vi "Create From String.vi"(8 "error in":errorcluster, 10 "Input String":string) -> (0 "error out":errorcluster, 3 "Orient3d out":refnum<class "Orient3d Class.lvclass">)   [LabVIEW 2011, in "Orient3d Class.lvclass"]
uses:
  Orient3d Class.lvclass
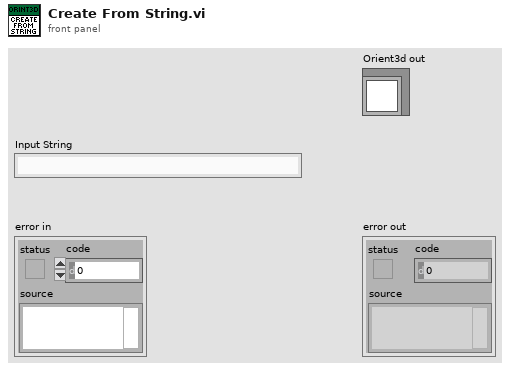
[diagram p1: front panel]
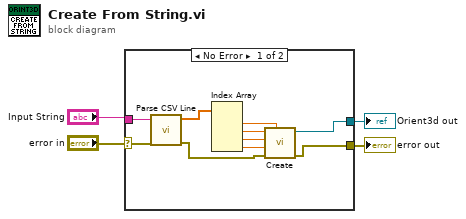
[diagram p0: block diagram]
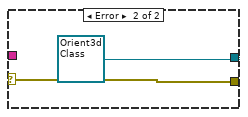
[diagram p2: hidden frame]
diagram:
  n1 = case shown="No Error" "error in" {
    selector: "error in" -> [w12 w16]
    tunnel: [w5 w16] -> w1
    tunnel: [w14 refnum<class "Orient3d Class.lvclass"> refnum ("Orient3d out")] -> w2
    tunnel: "Input String" -> [w13 _]
    frame No Error {
      n2 = call "Parse CSV Line.vi"("error in"=w12, "Input String"=w13) -> ("error out"=w6:errorcluster, "values"=w11:dbl[])  [unwired: 8 in]
      n3 = Index Array(array=w11) -> (element #1=w10:dbl, element #2=w9:dbl, element #3=w8:dbl, element #4=w7:dbl)  [unwired: 4 in]
      n4 = call "Create.vi"("x"=w10, "error in"=w6, "w"=w7, "z"=w8, "y"=w9) -> ("error out"=w5:errorcluster, "Orient3d out"=w14:refnum<class "Orient3d Class.lvclass">)  [unwired: 5 in]
    }
    frame Error {
    }
  }
  "error out" <- w1
  "Orient3d out" <- w2
